vi "WPI_CameraERRBadImageData.vi"() -> (0 "error out":errorcluster)   [LabVIEW 2017]
doc: "This software is licensed. Open the labview\\readme\\WPI Robotics Library Open Source License.txt file for more information."
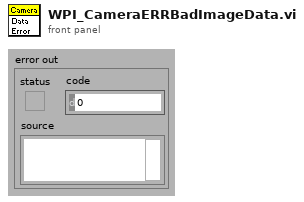
[diagram p1: front panel]
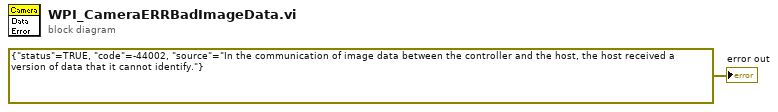
[diagram p0: block diagram]
diagram:
  "error out" <- errorcluster {"status"=TRUE, "code"=-44002, "source"="In the communication of image data between the controller and the host, the host received a version of data that it cannot identify."} ("error out 2")
